vi "SshKeepAlive.vi"(3 "SshShell":refnum<k24>, 7 "Pattern":string=">", 9 "error in (no error)":errorcluster) -> (0 "SshShell":refnum<k24>, 6 "error out":errorcluster)   [LabVIEW 2009]
uses:
  C:/Ohana/LV2009/OhanaOS-LV81/Instruments/Keyword/Controller/Tamir.sharpSsh.dll
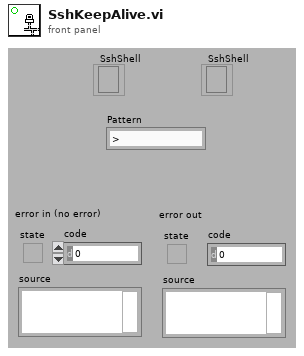
[diagram p1: front panel]
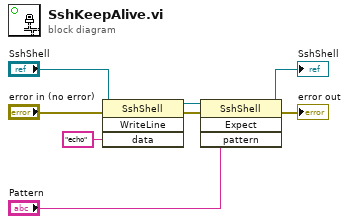
[diagram p0: block diagram]
diagram:
  n1 = invoke class="SshShell" method="WriteLine"(reference="SshShell", error in="error in (no error)", "data"="echo") -> (reference out=w2:refnum<k24>, error out=w3:errorcluster)  [unwired: 1 in, 2 out]
  n2 = invoke class="SshShell" method="Expect"(reference=w2, error in=w3, "pattern"="Pattern") -> (reference out=→"SshShell":refnum<k24>, error out=→"error out":errorcluster)  [unwired: 1 in, 2 out]
